vi "Pointer producer consumer TimeStampGenerator.vi"() -> (1 "TIME Numeric":ext, 2 "Local time (HHMMSS)":string, 3 "TIME hhmmss,units":fxp<+/-,64,32> format="%.3f")   [LabVIEW 2014]
panel:
  out "date/time string":string
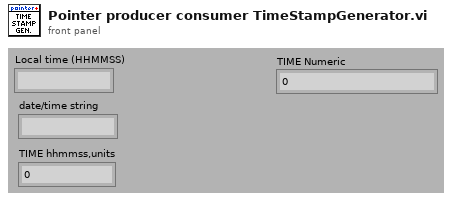
[diagram p1: front panel]
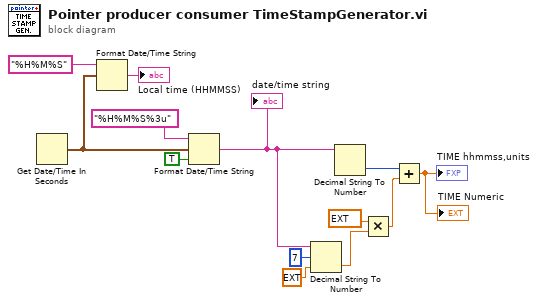
[diagram p0: block diagram]
diagram:
  n1 = Get Date/Time In Seconds() -> (seconds since 1Jan1904=w5:timestamp)
  n2 = Format Date/Time String(time format string (%c)="%H%M%S", seconds (now)=w5) -> (date/time string=→"Local time (HHMMSS)":string)  [unwired: 1 in]
  n3 = Format Date/Time String(time format string (%c)="%H%M%S%3u", seconds (now)=w5, UTC format=TRUE) -> (date/time string=w2:string)
  "date/time string" <- w2
  n4 = Decimal String To Number(string=w2, offset=7, default (0L)=ext 0.0 ("default (0 I32)")) -> (number=w10:ext)  [unwired: 1 out]
  n5 = Decimal String To Number(string=w2) -> (number=w12:i32)  [unwired: 2 in, 1 out]
  n6 = Multiply(x=ext 0.00099999999999999999996, y=w10) -> (x*y=w1:ext)
  n7 = Add(x=w12, y=w1) -> (x+y=→"TIME hhmmss,units" →"TIME Numeric":ext)
